vi "Activate-laser-measurement-hardware.vi"(8 "error in (no error)":errorcluster, 11 "SM1000-control in":T1) -> (0 "error out":errorcluster, 1 "Power":refnum<k21>, 2 "Control":refnum<k21>, 3 "SM1000-control out":T1, 4 "Batch size":i32, 5 "Timing":refnum<k21>)   [LabVIEW 2013, in "HardwareCharacterization.lvlib" / "HC-SM1000.lvclass"]
uses:
  HC-SM1000.lvclass
  Object-reference.ctl
  HC-SM1000.lvclass/HC-SM1000.ctl
  <vilib>/DAQmx/create/channels.llb/DAQmx Create Channel (AI-Voltage-Basic).vi
  <vilib>/DAQmx/create/channels.llb/DAQmx Create Channel (DI-Digital Input).vi
  <vilib>/DAQmx/configure/timing.llb/DAQmx Timing (Sample Clock).vi
  <vilib>/DAQmx/create/channels.llb/DAQmx Create Channel (CO-Pulse Generation-Frequency).vi
  <vilib>/DAQmx/configure/timing.llb/DAQmx Timing (Implicit).vi
  <resource>/objmgr/daqmx.rc
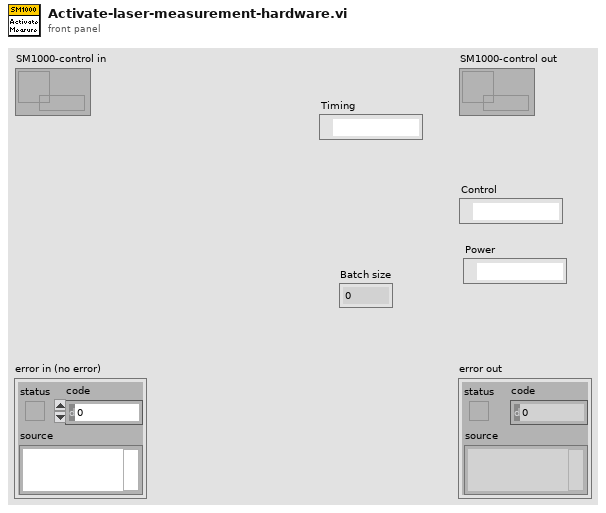
[diagram p1: front panel]
types:
  T1 = typedef "HardwareCharacterization.lvlib/HC-SM1000.lvclass/Object-reference.ctl" = refnum<data-value>
  T2 = typedef "HardwareCharacterization.lvlib/HC-SM1000.lvclass/Laser-response-settings.ctl" = cluster{"Timebase":tag, "Duty cycle":dbl, "Sample rate":dbl, "Batch size":i32, "Timing bypass":tag, "Modulation channel":tag, "Power channel":tag}
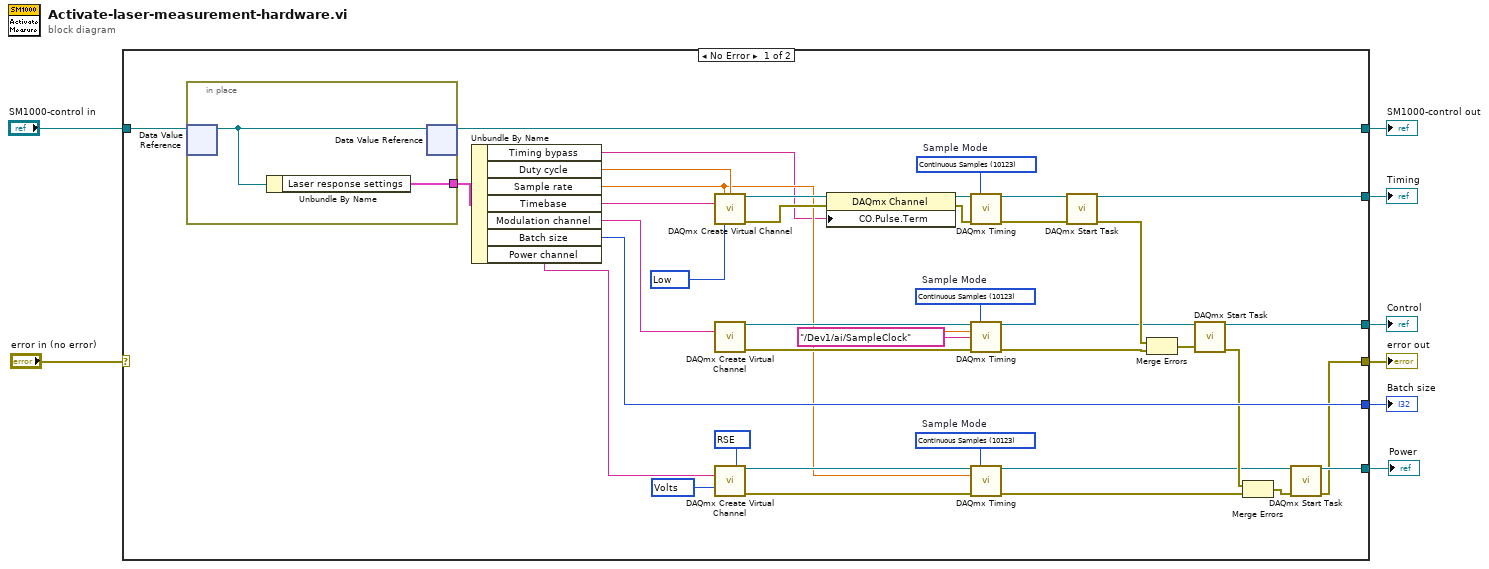
[diagram p0: block diagram]
diagram:
  n1 = case shown="No Error" "error in (no error)" {
    selector: "error in (no error)" -> [_ w51]
    tunnel: [w15 w51] -> w7
    tunnel: [w46 w50] -> w5
    tunnel: "SM1000-control in" -> [w47 w50]
    tunnel: [w14 _] -> w4
    tunnel: [w31 _] -> w3
    tunnel: [w28 _] -> w2
    tunnel: [w19 _] -> w1
    frame No Error {
      w23 = 10348 items=["Volts"=10348, "From Custom Scale"=10065] ("units")
      w24 = 10083 items=["default"=-1, "RSE"=10083, "NRSE"=10078, "Differential"=10106, "Pseudodifferential"=12529] ("input terminal configuration")
      w26 = 10123 items=["Finite Samples"=10178, "Continuous Samples"=10123, "Hardware Timed Single Point"=12522]  # Sample Mode
      w36 = 10123 items=["Finite Samples"=10178, "Continuous Samples"=10123, "Hardware Timed Single Point"=12522]  # Sample Mode
      w41 = 10123 items=["Finite Samples"=10178, "Continuous Samples"=10123, "Hardware Timed Single Point"=12522]  # Sample Mode
      w42 = 10214 items=["High"=10192, "Low"=10214] ("idle state")
      n2 = in-place {
        in-place-border: [w48] -> w45
        n3 = in-place-dvr #1(w47) -> (w49:refnum<class "HC-SM1000.lvclass">)  [unwired: 1 out]
        n4 = Unbundle By Name(w49) -> ("Laser response settings"=w48:T2)
        n5 = in-place-dvr #1(w49) -> (w46:T1)  [unwired: 1 out]
      }
      n6 = Unbundle By Name(w45) -> ("Timing bypass"=w20:tag, "Duty cycle"=w44:dbl, "Sample rate"=w21:dbl, "Timebase"=w43:tag, "Modulation channel"=w33:tag, "Batch size"=w28:i32, "Power channel"=w27:tag)
      n7 = call-poly <vilib>:"DAQmx Create Virtual Channel.vi"("frequency"=w21, "duty cycle"=w44, "counter"=w43, "idle state"=w42) -> ("task out"=w37:refnum<k21>, "error out"=w40:errorcluster)  [unwired: 10 in]
      n8 = call-poly <vilib>:"DAQmx Create Virtual Channel.vi"("lines"=w33) -> ("task out"=w35:refnum<k21>, "error out"=w34:errorcluster)  [unwired: 13 in]
      n9 = call-poly <vilib>:"DAQmx Create Virtual Channel.vi"("input terminal configuration"=w24, "physical channels"=w27, "units"=w23) -> ("task out"=w25:refnum<k21>, "error out"=w22:errorcluster)  [unwired: 11 in]
      n10 = property class="DAQmx Channel"(reference=w37, error in=w40, "CO.Pulse.Term"=w20) -> (reference out=w38:refnum<k21>, error out=w39:errorcluster)
      n11 = call-poly <vilib>:"DAQmx Timing.vi"("task/channels in"=w38, "sample mode"=w41, "error in"=w39) -> ("task out"=w32:refnum<k21>, "error out"=w30:errorcluster)  [unwired: 11 in]
      n12 = call-poly <vilib>:"DAQmx Timing.vi"("task/channels in"=w35, "sample mode"=w36, "rate"=w21, "source"=tag "/Dev1/ai/SampleClock", "error in"=w34) -> ("task out"=w9:refnum<k21>, "error out"=w10:errorcluster)  [unwired: 9 in]
      n13 = call-poly <vilib>:"DAQmx Timing.vi"("task/channels in"=w25, "sample mode"=w26, "rate"=w21, "error in"=w22) -> ("task out"=w12:refnum<k21>, "error out"=w11:errorcluster)  [unwired: 10 in]
      n14 = call <vilib>:"DAQmx Start Task.vi"("task/channels in"=w32, "error in"=w30) -> ("task out"=w31:refnum<k21>, "error out"=w29:errorcluster)  [unwired: 12 in]
      n15 = Merge Errors(w29, w10) -> (w18:errorcluster)
      n16 = call <vilib>:"DAQmx Start Task.vi"("task/channels in"=w9, "error in"=w18) -> ("task out"=w14:refnum<k21>, "error out"=w16:errorcluster)  [unwired: 12 in]
      n17 = Merge Errors(w16, w11) -> (w17:errorcluster)
      n18 = call <vilib>:"DAQmx Start Task.vi"("task/channels in"=w12, "error in"=w17) -> ("task out"=w19:refnum<k21>, "error out"=w15:errorcluster)  [unwired: 12 in]
    }
    frame Error {
    }
  }
  "error out" <- w7
  "SM1000-control out" <- w5
  "Control" <- w4
  "Timing" <- w3
  "Batch size" <- w2
  "Power" <- w1
